vi "StepWrite.vi"(7 "Cluster in":T2, 11 "error in":errorcluster) -> (8 "Results":T1, 15 "error out":errorcluster)   [LabVIEW 2021]
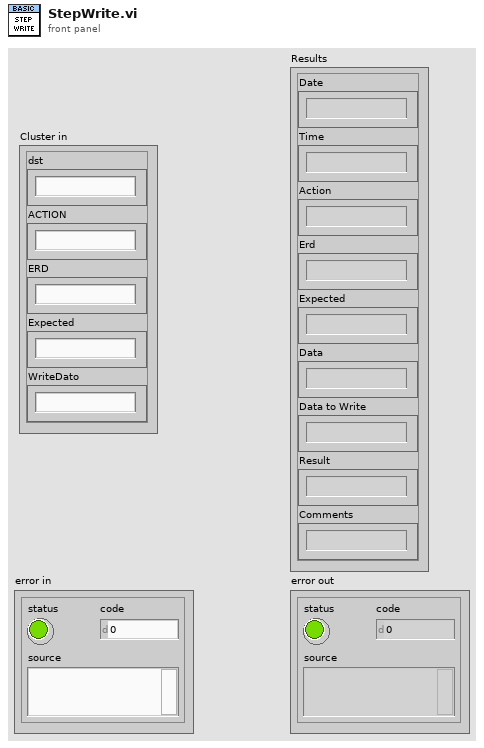
[diagram p1: front panel]
types:
  T1 = cluster{"Date":string, "Time":string, "Action":string, "Erd":string, "Expected":string, "Data":string, "Data to Write":string, "Result":string, "Comments":string}
  T2 = cluster{"dst":string, "ACTION":string, "ERD":string, "Expected":string, "WriteDato":string}
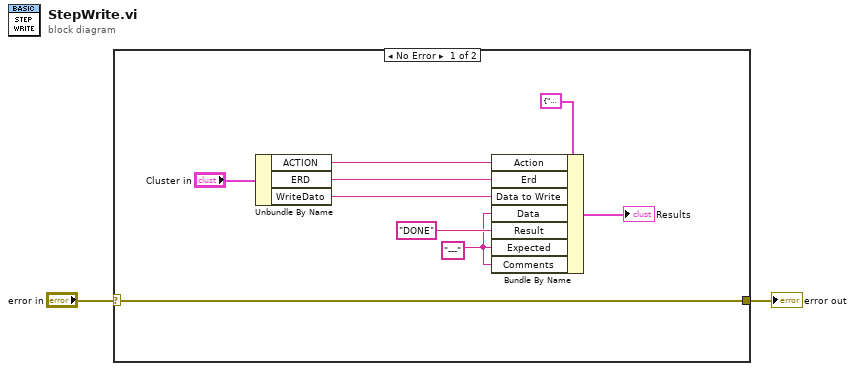
[diagram p0: block diagram]
diagram:
  n1 = case shown="No Error" "error in" {
    selector: "error in" -> [w3 w12]
    tunnel: [w3 w12] -> w1
    frame No Error {
      w4 = "---"
      n2 = Unbundle By Name("Cluster in") -> ("ACTION"=w9:string, "ERD"=w8:string, "WriteDato"=w7:string)
      n3 = Bundle By Name(cluster=T1 {"Date"="", "Time"="", "Action"="", "Erd"="", "Expected"="", "Data"="", "Data to Write"="", "Result"="", "Comments"=""}, "Action"=w9, "Erd"=w8, "Data to Write"=w7, "Data"=w4, "Result"="DONE", "Expected"=w4, "Comments"=w4) -> (→"Results":T1)
    }
    frame Error {
    }
  }
  "error out" <- w1
